vi "RangeMin_Write.vi"(4 "error in (no error)":errorcluster, 5 "Value":dbl, 6 "Container State":T2, 7 "Display State In":T1) -> (0 "error out":errorcluster, 3 "Display State Out":T1)   [LabVIEW 2012, in "Time Slider.xctl"]
uses:
  Time Slider.xctl
  <vilib>/_xctls/Container State.ctl
  Timing State.ctl
  <vilib>/_xctls/XControlSupport.lvlib
panel:
  # "Replace the Value Control below with a Control of desired type.\nDo not remove this Control or the others from the connector pane.\nDo not change the connector pane pattern.\nThe Value control should always be the third terminal from top on the input side in the connector pane."
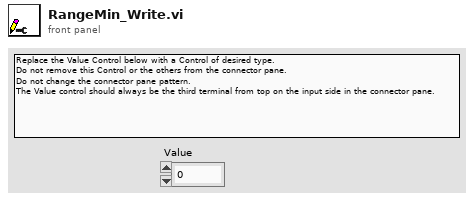
[diagram p1: front panel]
types:
  T1 = typedef "Time Slider.xctl/Timing State.ctl" = cluster{"Range Max":dbl, "Range Min":dbl}
  T2 = typedef "XControlSupport.lvlib/Container State.ctl" = cluster{"Indicator?":bool, "Run Mode?":bool, " Refnum":refnum<vi>}
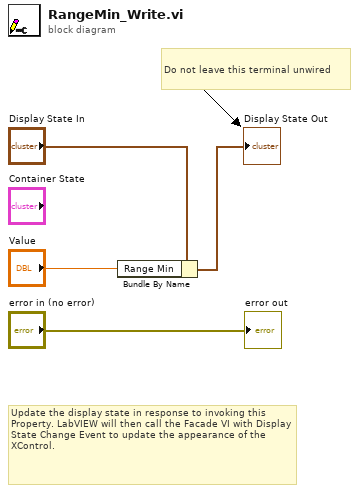
[diagram p0: block diagram]
diagram:
  # "Do not leave this terminal unwired"
  # "Update the display state in response to invoking this Property. LabVIEW will then call the Facade VI with Display State Change Event to update the appearance of the XControl."
  n1 = Bundle By Name(cluster="Display State In", "Range Min"="Value") -> (→"Display State Out":T1)
  "error out" <- "error in (no error)"
